vi "TLPM_PowerMeter_Open.vi"() -> (0 "error out":errorcluster {"code" format="%.0x"}, 3 "instrument handle out":refnum<visa-resource-name>)   [LabVIEW 2014]
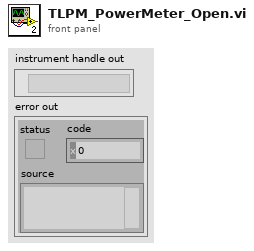
[diagram p1: front panel]
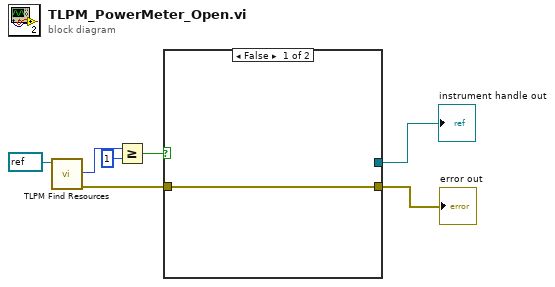
[diagram p0: block diagram]
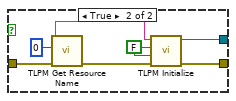
[diagram p2: hidden frame]
diagram:
  n1 = call "TLPM Find Resources.vi"("instrument handle"=refnum<visa-resource-name> refnum) -> ("error out"=w1:errorcluster, "Resource Count"=w6:u32)  [unwired: 8 in, 1 out]
  n2 = Greater Or Equal?(x=w6, y=u32 1) -> (x >= y?=w2:bool)
  n3 = case shown="False" w2 {
    tunnel: [_ w11] -> w4
    tunnel: [w8 w10] -> w3
    tunnel: w1 -> [w8 w9]
    frame False {
    }
    frame True {
      w12 = FALSE ("ID Query (Do Query)")
      n4 = call "TLPM Get Resource Name.vi"("error in (no error)"=w9, "Index (0)"=u32 0 ("Device Index")) -> ("error out"=w15:errorcluster, "Resource Name"=w14:string)  [unwired: 7 in, 1 out]
      n5 = call "TLPM Initialize.vi"("error in (no error)"=w15, "Reset Device (Reset Device)"=w12, "ID Query (Do Query)"=w12, "resource name"=w14) -> ("error out"=w10:errorcluster, "instrument handle out"=w11:refnum<visa-resource-name>)  [unwired: 6 in]
    }
  }
  "instrument handle out" <- w4
  "error out" <- w3
